vi "Config.vi"(8 "error in (no error)":errorcluster, 10 "Setting":variant, 11 "NI Scope in":refnum<class "NI Scope.lvclass">) -> (0 "error out":errorcluster, 3 "NI Scope out":refnum<class "NI Scope.lvclass">)   [LabVIEW 2025, in "Scope.lvlib" / "NI Scope.lvclass"]
uses:
  NI Scope.lvclass
  C:/Users/Public/Documents/Sandia National Labs/TSS Plugin/CEF.lvlibp/Node/CEF_Node.lvclass
  C:/Working copy/tss/Plugin/Engines/Scope/Scope Instrument/Scope Instrument.lvclass
  C:/Users/Public/Documents/Sandia National Labs/TSS Plugin/Abstract Engine.lvlibp/Abstract Instrument/Abstract Instrument.lvclass
  Scope Channel/Scope Channel.lvclass
  Scope configuration/Scope configuration.lvclass
  C:/Users/Public/Documents/Sandia National Labs/TSS Plugin/Abstract Engine.lvlibp/Instrument configuration/Instrument configuration.lvclass
  NI Scope.lvclass/NI Scope.ctl
  Scope configuration/Scope configuration.lvclass/Scope configuration.ctl
  <instrlib>/niScope/Controls/niScope trigger coupling.ctl
  Users/Public/Documents/Sandia National Labs/TSS Plugin/Abstract Engine.lvlibp/Abstract Instrument/Channel.ctl
  Scope Channel configuration/Scope Channel configuration.lvclass
  C:/Users/Public/Documents/Sandia National Labs/TSS Plugin/Abstract Engine.lvlibp/Channel configuration/Channel configuration.lvclass
  Scope Channel configuration/Scope Channel configuration.lvclass/Scope Channel configuration.ctl
  <instrlib>/niScope/Controls/niScope vertical coupling.ctl
  <instrlib>/niScope/Controls/niScope trigger slope.ctl
  <instrlib>/niScope/Controls/niScope trigger window mode.ctl
  Scope Channel configuration/Read Scope Channel.vi
  Scope configuration/Read Scope Setting.vi
  Users/Public/Documents/Sandia National Labs/TSS Plugin/CEF.lvlibp/Node/ReadChildren.vi
  Users/Public/Documents/Sandia National Labs/TSS Plugin/Abstract Engine.lvlibp/Instrument configuration/Read Instrument Setting.vi
  Users/Public/Documents/Sandia National Labs/TSS Plugin/Abstract Engine.lvlibp/Channel configuration/Read Channel Setting.vi
  <instrlib>/niScope/Configure/Trigger/niScope Configure Trigger Edge.vi
  <instrlib>/niScope/Configure/Trigger/niScope Configure Trigger Digital.vi
  Users/Public/Documents/Sandia National Labs/TSS Plugin/CEF.lvlibp/Node/CEF_Node.lvclass
  Users/Public/Documents/Sandia National Labs/TSS Plugin/CEF.lvlibp/serializable configuration/CEF_serializable configuration.lvclass
  Users/Public/Documents/Sandia National Labs/TSS Plugin/Abstract Engine.lvlibp/Abstract Instrument/Abstract Instrument.lvclass
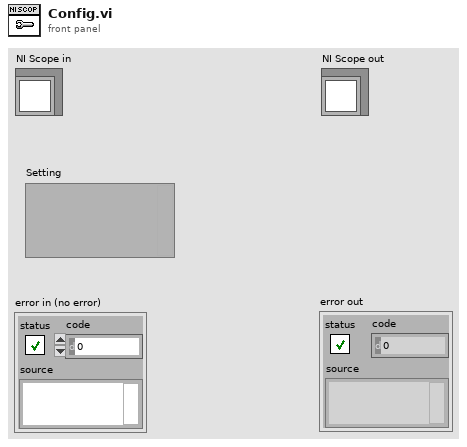
[diagram p1: front panel]
types:
  T1 = typedef "Abstract Engine.lvlibp/Instrument configuration.lvclass/Default Instrument.ctl" = cluster{"Type":string, "Address":string, "SW Alias":string, "Description":string, "Enabled":bool}
  T2 = typedef "Scope.lvlib/Scope configuration.lvclass/Scope Instrument Setting.ctl" = cluster{"Sampling Rate":dbl, "Number of Samples":u32, "Type":string, "Pretrigger":dbl, "Source":string, "Level 1":dbl, "Level 2":dbl, "Trigger Coupling":string, "TrigDest":string, "Group":string}
  T3 = typedef "Abstract Engine.lvlibp/Abstract Instrument.lvclass/Channel.ctl" = cluster{"Alias":string, "DataType":enum16{"Anaolg Input", "Waveform"}, "Unit":enum16{"---", "V", "A", "Ohm", "Hz", "uF", "degC", "deg"}, "Upper limit":dbl, "Lower limit":dbl, "Measurement":variant}
  T4 = typedef "niScope trigger coupling.ctl" = u16
  T5 = typedef "Abstract Engine.lvlibp/Channel configuration.lvclass/Default Channel.ctl" = cluster{"Address":string, "SW Alias":string, "Enabled":bool, "Type":string, "Description":string}
  T6 = typedef "Scope.lvlib/Scope Channel configuration.lvclass/Scope Channel Setting.ctl" = cluster{"Gain":u32, "Offset":u32, "Vertical Range":dbl, "Vertical Offset":dbl, "Unit":string, "Attenuation":dbl, "Vertical Coupling":string, "Impedance":string, "Auto Setup":bool}
  T7 = typedef "niScope vertical coupling.ctl" = i32
  T8 = typedef "niScope trigger slope.ctl" = i32
  T9 = typedef "niScope trigger window mode.ctl" = i32
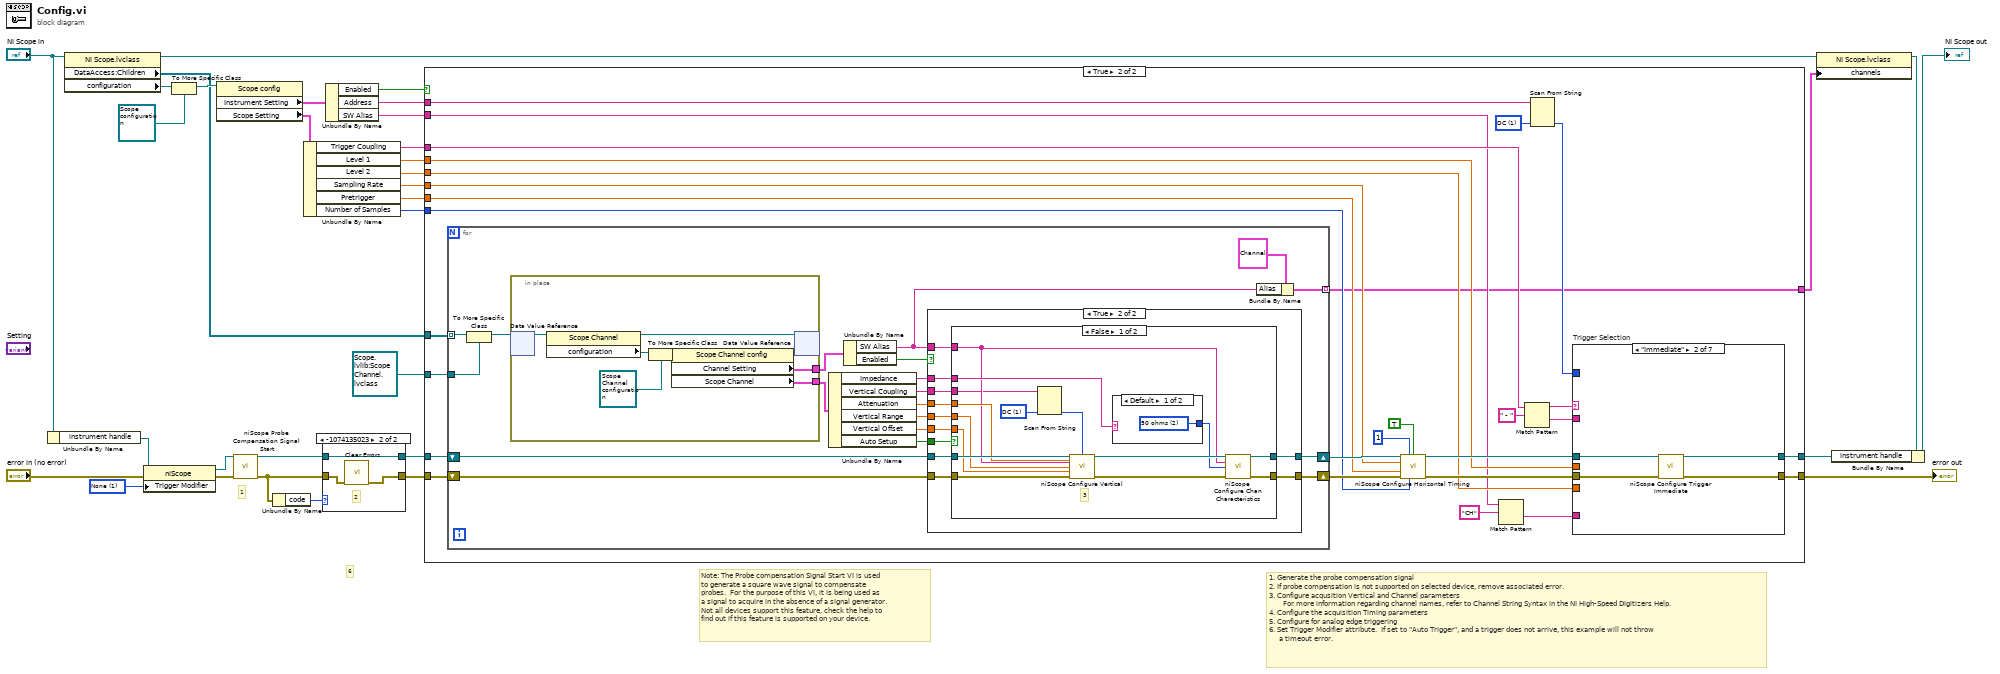
[diagram p0: block diagram]
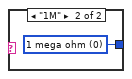
[diagram p4: hidden frame]
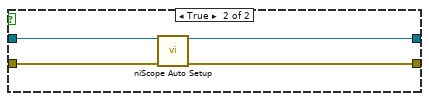
[diagram p5: hidden frame]
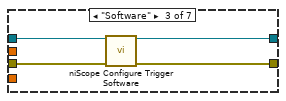
[diagram p7: hidden frame]
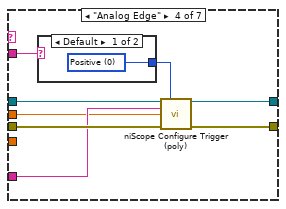
[diagram p8: hidden frame]
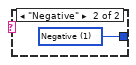
[diagram p9: hidden frame]
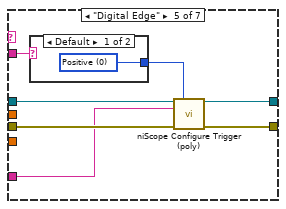
[diagram p10: hidden frame]
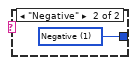
[diagram p11: hidden frame]
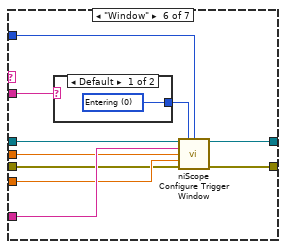
[diagram p12: hidden frame]
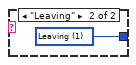
[diagram p13: hidden frame]
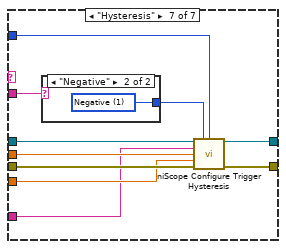
[diagram p14: hidden frame]
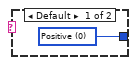
[diagram p15: hidden frame]
diagram:
  w32 = 1 items=["None"=1, "Auto Trigger"=2] ("Triggering:Trigger Modifier")
  # "1"
  # "Note: The Probe compensation Signal Start VI is used\nto generate a square wave signal to compensate\nprobes.  For the purpose of this VI, it is being used as\na signal to acquire in the absence of a signal generator.\nNot all devices support this feature, check the help to\nfind out if this feature is supported on your device."
  # "1. Generate the probe compensation signal \n2. If probe compensation is not supported on selected device, remove associated error.\n3. Configure acqusition Vertical and Channel parameters\n       For more information regarding channel names, refer to Channel String Syntax in the NI High-Speed Digitizers Help.\n4. Configure the acquisition Timing parameters\n5. Configure for analog edge triggering\n6. Set Trigger Modifier attribute.  If set to \"Auto Trigger\", and a trigger does not arrive, this example will not throw\n     a timeout error."
  # "6"
  n1 = Unbundle By Name("NI Scope in") -> ("instrument handle"=w4:refnum<k15>)
  n2 = property class="NI Scope.lvclass"(reference="NI Scope in") -> (reference out=w31:refnum<class "NI Scope.lvclass">, "DataAccess:Children"=w24:refnum<data-value>[], "configuration"=w29:refnum<class "CEF_serializable configuration.lvclass">)  [unwired: 1 in, 1 out]
  n3 = property class="niScope"(reference=w4, error in="error in (no error)", "Trigger Modifier"=w32) -> (reference out=w3:refnum<k15>, error out=w5:errorcluster)
  n4 = To More Specific Class(target class=refnum<class "Scope configuration.lvclass"> refnum ("Scope.lvlib:Scope configuration.lvclass"), reference=w29) -> (specific class reference=w28:refnum<class "Scope configuration.lvclass">)  [unwired: 1 in, 1 out]
  n5 = property class="Scope config"(reference=w28) -> ("Instrument Setting"=w26:T1, "Scope Setting"=w15:T2)  [unwired: 1 in, 2 out]
  n6 = call <instrlib>:"niScope Probe Compensation Signal Start.vi"("instrument handle"=w3, "error in"=w5) -> ("instrument handle out"=w20:refnum<k15>, "error out"=w19:errorcluster)  [unwired: 12 in]
  n7 = Unbundle By Name(w19) -> ("code"=w21:i32)
  n8 = Unbundle By Name(w15) -> ("Trigger Coupling"=w9:string, "Level 1"=w14:dbl, "Level 2"=w13:dbl, "Sampling Rate"=w12:dbl, "Pretrigger"=w11:dbl, "Number of Samples"=w10:u32)
  n9 = case shown="-1074135023" w21 {
    tunnel: [w34 w38] -> w18
    tunnel: w20 -> [w35 w36]
    tunnel: [w35 w36] -> w17
    tunnel: w19 -> [w34 w37]
    frame 0, Default {
    }
    frame -1074135023 {
      # "2"
      n10 = call <vilib>:"Clear Errors.vi"("error in (no error)"=w37) -> ("error out"=w38:errorcluster)  [unwired: 5 in, 1 out]
    }
  }
  n11 = Unbundle By Name(w26) -> ("Enabled"=w25:bool, "Address"=w22:string, "SW Alias"=w16:string)
  n12 = case shown="True" w25 {
    tunnel: w24 -> [_ w68]
    tunnel: refnum<data-value> refnum ("data value reference") -> [_ w67]
    tunnel: w9 -> [_ w61]
    tunnel: w22 -> [_ w47]
    tunnel: w18 -> [w40 w66]
    tunnel: w17 -> [w39 w65]
    tunnel: w10 -> [_ w56]
    tunnel: w12 -> [_ w53]
    tunnel: w11 -> [_ w52]
    tunnel: w16 -> [_ w44]
    tunnel: w14 -> [_ w51]
    tunnel: w13 -> [_ w50]
    tunnel: [w40 w49] -> w7
    tunnel: [w39 w48] -> w8
    tunnel: [_ w41] -> w1
    frame False {
    }
    frame True {
      w46 = T4 1 items=["AC"=0, "DC"=1, "HF Reject"=3, "LF Reject"=4, "AC Plus HF Reject"=1001] ("trigger coupling")
      n13 = for {
        tunnel: w68 -> [w86] mode=indexing
        tunnel: w67 -> [w85]
        shift-right: [w82] -> w60
        shift-left: w66 -> [w84]
        shift-right: [w81] -> w59
        shift-left: w65 -> [w83]
        tunnel: [w70] -> w41 mode=indexing
        n14 = To More Specific Class(target class=w85, reference=w86) -> (specific class reference=w87:refnum<data-value>)  [unwired: 1 in, 1 out]
        n15 = in-place {
          in-place-border: [w92] -> w80
          in-place-border: [w88] -> w79
          # "Initialize the front panel controls when loaded"
          n16 = in-place-dvr #1(w87) -> (w94:refnum<class "Scope Channel.lvclass">)  [unwired: 1 out]
          n17 = property class="Scope Channel"(reference=w94) -> (reference out=w93:refnum<class "Scope Channel.lvclass">, "configuration"=w91:refnum<class "CEF_serializable configuration.lvclass">)  [unwired: 1 in, 1 out]
          n18 = To More Specific Class(target class=refnum<class "Scope Channel configuration.lvclass"> refnum ("Scope.lvlib:Scope Channel configuration.lvclass"), reference=w91) -> (specific class reference=w90:refnum<class "Scope Channel configuration.lvclass">)  [unwired: 1 in, 1 out]
          n19 = property class="Scope Channel config"(reference=w90) -> ("Channel Setting"=w92:T5, "Scope Channel"=w88:T6)  [unwired: 1 in, 2 out]
          n20 = in-place-dvr #1(w93) -> ()  [unwired: 2 out]
        }
        n21 = Unbundle By Name(w79) -> ("Impedance"=w78:string, "Vertical Coupling"=w77:string, "Attenuation"=w76:dbl, "Vertical Range"=w75:dbl, "Vertical Offset"=w74:dbl, "Auto Setup"=w73:bool)
        n22 = Unbundle By Name(w80) -> ("SW Alias"=w71:string, "Enabled"=w72:bool)
        n23 = case shown="True" w72 {
          tunnel: w84 -> [w96 w107]
          tunnel: w73 -> [_ w106]
          tunnel: w83 -> [w95 w105]
          tunnel: [w96 w104] -> w82
          tunnel: w71 -> [_ w103]
          tunnel: w75 -> [_ w102]
          tunnel: w74 -> [_ w101]
          tunnel: w76 -> [_ w100]
          tunnel: w77 -> [_ w99]
          tunnel: w78 -> [_ w98]
          tunnel: [w95 w97] -> w81
          frame False {
          }
          frame True {
            n24 = case shown="False" w106 {
              tunnel: w107 -> [w120 w128]
              tunnel: w105 -> [w119 w127]
              tunnel: [w112 w126] -> w104
              tunnel: [w118 w125] -> w97
              tunnel: w103 -> [w111 _]
              tunnel: w102 -> [w117 _]
              tunnel: w101 -> [w116 _]
              tunnel: w100 -> [w115 _]
              tunnel: w99 -> [w109 _]
              tunnel: w98 -> [w114 _]
              frame False {
                w110 = T7 1 items=["AC", "DC", "Ground"] ("vertical coupling")
                # "3"
                n25 = Scan From String(input string=w109, default 1=w110) -> (output 1=w108:T7)  [unwired: 3 in, 3 out]
                n26 = call <instrlib>:"niScope Configure Vertical.vi"("instrument handle"=w119, "probe attenuation"=w115, "vertical coupling"=w108, "channels"=w111, "vertical range"=w117, "vertical offset"=w116, "error in"=w120) -> ("instrument handle out"=w122:refnum<k15>, "error out"=w121:errorcluster)  [unwired: 7 in]
                n27 = case shown="Default" w114 {
                  tunnel: [w123 w124] -> w113
                  frame Default {
                    w123 = u32 2 items=["1 mega ohm"=0, "50 ohms"=2] ("input impedance")
                  }
                  frame "1M" {
                    w124 = u32 0 items=["1 mega ohm"=0, "50 ohms"=2] ("input impedance")
                  }
                }
                n28 = call <instrlib>:"niScope Configure Chan Characteristics.vi"("instrument handle"=w122, "channels"=w111, "input impedance"=w113, "error in"=w121) -> ("instrument handle out"=w118:refnum<k15>, "error out"=w112:errorcluster)  [unwired: 10 in]
              }
              frame True {
                n29 = call <instrlib>:"niScope Auto Setup.vi"("instrument handle"=w127, "error in"=w128) -> ("instrument handle out"=w125:refnum<k15>, "error out"=w126:errorcluster)  [unwired: 12 in]
              }
            }
          }
        }
        n30 = Bundle By Name(cluster=T3 {"Alias"="ch0", "DataType"=enum."Anaolg Input", "Unit"=enum."V", "Upper limit"=10.0, "Lower limit"=-10.0, "Measurement"=variant} ("Channel"), "Alias"=w71) -> (w70:T3)
      }
      n31 = call <instrlib>:"niScope Configure Horizontal Timing.vi"("instrument handle"=w59, "number of records"=1, "enforce realtime"=TRUE, "min sample rate"=w53, "reference position"=w52, "error in"=w60, "min record length"=w56) -> ("instrument handle out"=w57:refnum<k15>, "error out"=w58:errorcluster)  [unwired: 7 in]
      n32 = Match Pattern(string=w44, regular expression="CH") -> (after substring=w42:string)  [unwired: 1 in, 3 out]
      n33 = Match Pattern(string=w61, regular expression=" - ") -> (before substring=w64:string, after substring=w63:string)  [unwired: 1 in, 2 out]
      n34 = Scan From String(input string=w47, default 1=w46) -> (output 1=w45:T4)  [unwired: 3 in, 3 out]
      n35 = case "Trigger Selection" shown="\"Immediate\"" w64 {
        tunnel: [w129 w131 w135 w143 w151 w160 w177] -> w49
        tunnel: [w130 w133 w137 w141 w153 w159 w175] -> w48
        tunnel: w63 -> [_ _ _ w146 w155 w167 w179]
        tunnel: w57 -> [w130 w134 w138 w142 w154 w166 w176]
        tunnel: w58 -> [w129 w132 w136 w144 w152 w162 w178]
        tunnel: w42 -> [_ _ _ w140 w149 w165 w170]
        tunnel: w51 -> [_ _ _ w139 _ w164 w172]
        tunnel: w50 -> [_ _ _ _ _ w163 w171]
        tunnel: w45 -> [_ _ _ _ _ w158 w173]
        frame Default {
        }
        frame "Immediate" {
          n36 = call <instrlib>:"niScope Configure Trigger Immediate.vi"("instrument handle"=w134, "error in"=w132) -> ("instrument handle out"=w133:refnum<k15>, "error out"=w131:errorcluster)  [unwired: 12 in]
        }
        frame "Software" {
          n37 = call <instrlib>:"niScope Configure Trigger Software.vi"("instrument handle"=w138, "error in"=w136) -> ("instrument handle out"=w137:refnum<k15>, "error out"=w135:errorcluster)  [unwired: 12 in]
        }
        frame "Analog Edge" {
          n38 = case shown="Default" w146 {
            tunnel: [w147 w148] -> w145
            frame Default {
              w147 = T8 0 items=["Positive", "Negative"] ("trigger slope")
            }
            frame "Negative" {
              w148 = T8 1 items=["Positive", "Negative"] ("trigger slope")
            }
          }
          n39 = call-poly <instrlib>:"niScope Configure Trigger (poly).vi"("instrument handle"=w142, "trigger slope"=w145, "trigger source"=w140, "trigger level"=w139, "error in"=w144) -> ("instrument handle out"=w141:refnum<k15>, "error out"=w143:errorcluster)  [unwired: 9 in]
        }
        frame "Digital Edge" {
          n40 = case shown="Default" w155 {
            tunnel: [w156 w157] -> w150
            frame Default {
              w156 = T8 0 items=["Positive", "Negative"] ("trigger slope")
            }
            frame "Negative" {
              w157 = T8 1 items=["Positive", "Negative"] ("trigger slope")
            }
          }
          n41 = call-poly <instrlib>:"niScope Configure Trigger (poly).vi"("instrument handle"=w154, "trigger slope"=w150, "trigger source"=w149, "error in"=w152) -> ("instrument handle out"=w153:refnum<k15>, "error out"=w151:errorcluster)  [unwired: 10 in]
        }
        frame "Window" {
          n42 = case shown="Default" w167 {
            tunnel: [w168 w169] -> w161
            frame Default {
              w168 = T9 0 items=["Entering", "Leaving"] ("trigger window mode")
            }
            frame "Leaving" {
              w169 = T9 1 items=["Entering", "Leaving"] ("trigger window mode")
            }
          }
          n43 = call <instrlib>:"niScope Configure Trigger Window.vi"("instrument handle"=w166, "trigger window mode"=w161, "trigger coupling"=w158, "trigger source"=w165, "low level"=w164, "high level"=w163, "error in"=w162) -> ("instrument handle out"=w159:refnum<k15>, "error out"=w160:errorcluster)  [unwired: 7 in]
        }
        frame "Hysteresis" {
          n44 = case shown="\"Negative\"" w179 {
            tunnel: [w180 w181] -> w174
            frame Default {
              w180 = T8 0 items=["Positive", "Negative"] ("trigger slope")
            }
            frame "Negative" {
              w181 = T8 1 items=["Positive", "Negative"] ("trigger slope")
            }
          }
          n45 = call <instrlib>:"niScope Configure Trigger Hysteresis.vi"("instrument handle"=w176, "trigger slope"=w174, "trigger coupling"=w173, "trigger source"=w170, "trigger level"=w172, "hysteresis"=w171, "error in"=w178) -> ("instrument handle out"=w175:refnum<k15>, "error out"=w177:errorcluster)  [unwired: 7 in]
        }
      }
    }
  }
  "error out" <- w7
  n46 = property class="NI Scope.lvclass"(reference=w31, "channels"=w1) -> (reference out=w2:refnum<class "NI Scope.lvclass">)  [unwired: 1 in, 1 out]
  n47 = Bundle By Name(cluster=w2, "instrument handle"=w8) -> (→"NI Scope out":refnum<class "NI Scope.lvclass">)
